vi "dfd_FXP Cascaded SOS Form I with IS.vi"(6 "state in":i64[](array[numeric]), 7 "quantizers":T5[](array[typedef]) {"source" items=["Coef a/k"=0, "Coef b/v"=7, "Input"=1, "Output"=2, "Multiplicand"=3, "Product"=4, "Sum"=5, "Delay"=6, "Gain"=8]}, 8 "filtering statistics in":T4(array[cluster]) {"statistics information"."min value" format="%.2f"; "statistics information"."max value" format="%.2f"; "Quantizer Source" items=["Coefficients a/k"=0, "Coefficients b/v"=7, "Input"=1, "Output"=2, "Multiplicand"=3, "Product"=4, "Sum"=5, "Delay"=6]}, 9 "coef a":T7, 10 "coef b":T7, 11 "X":T7) -> (0 "filtering statistics out":T4(array[cluster]) {"statistics information"."min value" format="%.2f"; "statistics information"."max value" format="%.2f"; "Quantizer Source" items=["Coefficients a/k"=0, "Coefficients b/v"=7, "Input"=1, "Output"=2, "Multiplicand"=3, "Product"=4, "Sum"=5, "Delay"=6]}, 3 "filtered X":T7, 4 "state out":i64[](array[numeric]))   [LabVIEW 2017, in "NI_DigFilter_FXP.lvlib"]
uses:
  <vilib>/addons/Digital Filter Design/NI_DigFilter_FXP.lvlib
  <vilib>/addons/Digital Filter Design/_Objects.llb/dfd_DFXP Data Type (vector).ctl
  <vilib>/addons/Digital Filter Design/_Objects.llb/dfd_DFXP Operation Parameter.ctl
  <vilib>/addons/Digital Filter Design/_Objects.llb/dfd_Internal Quantization Srcs.ctl
  <vilib>/addons/Digital Filter Design/_Objects.llb/DFD Quantization Sources.ctl
  <vilib>/addons/Digital Filter Design/_Objects.llb/DFD FXP Statistics Data.ctl
  <vilib>/addons/Digital Filter Design/_Objects.llb/dfd_DFXP Data Type (scaler).ctl
  <vilib>/addons/Digital Filter Design/NI_DigFilterLicensed.lvlib
panel:
  in  "DFXP Value":T1={"value"=0, "wl"=0, "iwl"=0, "Signed"=TRUE} {"value" format="%.0x"}
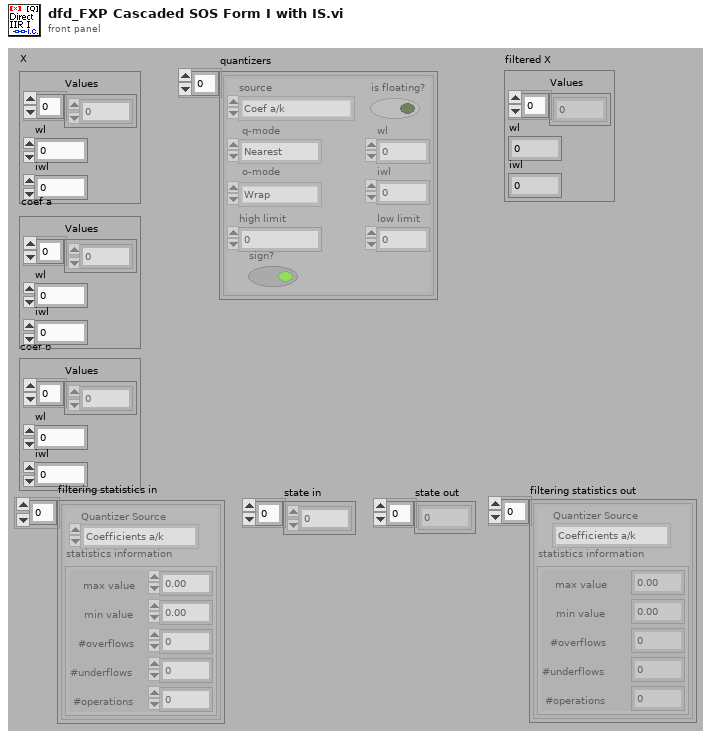
[diagram p1: front panel]
types:
  T1 = typedef "dfd_DFXP Data Type (scaler).ctl" = cluster{"value":i64, "wl":i16, "iwl":i16, "Signed":bool}
  T2 = typedef "NI_DigFilterLicensed.lvlib/DFD Quantization Sources.ctl" = u16
  T3 = typedef "NI_DigFilterLicensed.lvlib/DFD FXP Statistics Data.ctl" = cluster{"max value":ext, "min value":ext, "#overflows":i32, "#underflows":i32, "#operations":i32}
  T4 = cluster{"Quantizer Source":T2, "statistics information":T3}[]
  T5 = typedef "dfd_DFXP Operation Parameter.ctl" = cluster{"source":T6, "is floating?":bool, "o-mode":enum16{"Saturation", "Wrap"}, "q-mode":enum16{"Nearest", "Truncation"}, "wl":i16, "high limit":i64, "low limit":i64, "iwl":i16, "sign?":bool}
  T6 = typedef "NI_DigFilterLicensed.lvlib/dfd_Internal Quantization Srcs.ctl" = u16
  T7 = typedef "dfd_DFXP Data Type (vector).ctl" = cluster{"Values":i64[], "wl":i16, "iwl":i16}
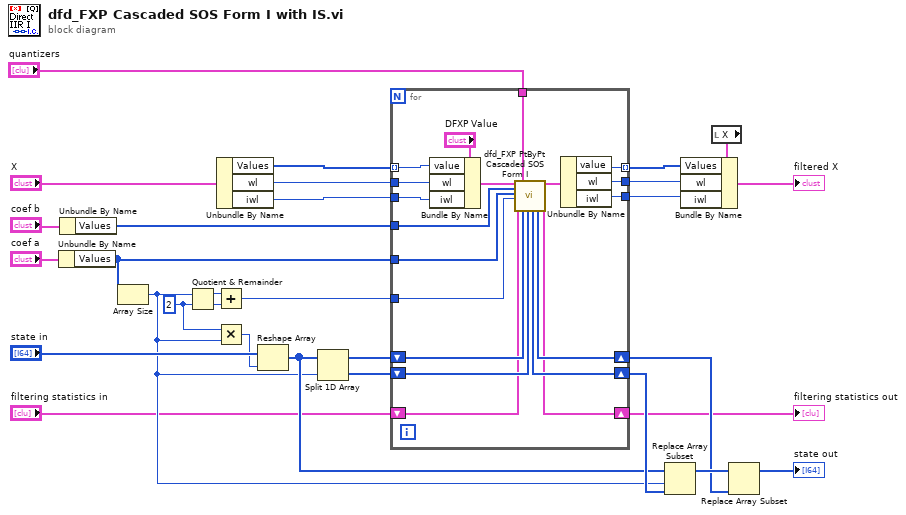
[diagram p0: block diagram]
diagram:
  w25 = 2 ("y")
  n1 = Unbundle By Name("coef a") -> ("Values"=w8:i64[])
  n2 = Unbundle By Name("coef b") -> ("Values"=w9:i64[])
  n3 = Array Size(array=w8) -> (size(s)=w15:i32)
  n4 = Quotient & Remainder(x=w15, y=w25) -> (x-y*floor(x/y)=w30:i32, floor(x/y)=w29:i32)
  n5 = Add(x=w30, y=w29) -> (x+y=w27:i32)
  n6 = Multiply(x=w25, y=w15) -> (x*y=w23:i32)
  n7 = Unbundle By Name("X") -> ("Values"=w7:i64[], "wl"=w6:i16, "iwl"=w5:i16)
  n8 = Reshape Array("state in", w23) -> (w16:i64[])
  n9 = Split 1D Array(array=w16, index=w15) -> (first subarray=w22:i64[], second subarray=w21:i64[])
  n10 = for {
    tunnel: w7 -> [w49] mode=indexing
    shift-right: [w42] -> w13
    shift-left: w22 -> [w45]
    tunnel: w9 -> [w48]
    tunnel: w27 -> [w47]
    shift-right: [w43] -> w17
    shift-left: w21 -> [w44]
    tunnel: w8 -> [w46]
    tunnel: [w33] -> w18 mode=indexing
    tunnel: "quantizers" -> [w40]
    shift-right: [w38] -> w10
    shift-left: "filtering statistics in" -> [w39]
    tunnel: w6 -> [w35]
    tunnel: w5 -> [w34]
    tunnel: [w32] -> w2
    tunnel: [w31] -> w1
    n11 = Bundle By Name(cluster="DFXP Value", "value"=w49, "wl"=w35, "iwl"=w34) -> (w37:T1)
    n12 = call <vilib>:"dfd_FXP PtByPt Cascaded SOS Form I.vi"("x"=w37, "coef b"=w48, "coef a"=w46, "#sec"=w47, "filtering statistics in"=w39, "quantizers"=w40, "xState in"=w45, "yState in"=w44) -> ("yState out"=w43:i64[], "xState out"=w42:i64[], "filtered x"=w41:T1, "filtering statistics out"=w38:T4)  [unwired: 8 out]
    n13 = Unbundle By Name(w41) -> ("value"=w33:i64, "wl"=w32:i16, "iwl"=w31:i16)
  }
  "filtering statistics out" <- w10
  n14 = Replace Array Subset(array=w16, new element=w17, index=w15) -> (w14:i64[])
  n15 = local read "X"() -> (w3:T7)
  n16 = Bundle By Name(cluster=w3, "Values"=w18, "wl"=w2, "iwl"=w1) -> (→"filtered X":T7)
  n17 = Replace Array Subset(array=w14, new element=w13) -> (→"state out":i64[])  [unwired: 1 in]
